vi "PushClosedSet.vi"(9 "Novo nó":dbl[](array[numeric]), 10 "ClosedSet":dbl[][](array[numeric])) -> (2 "NewClosedSet":dbl[][](array[numeric]))   [LabVIEW 2016]
panel:
  # "x"
  # "id"
  # "y"
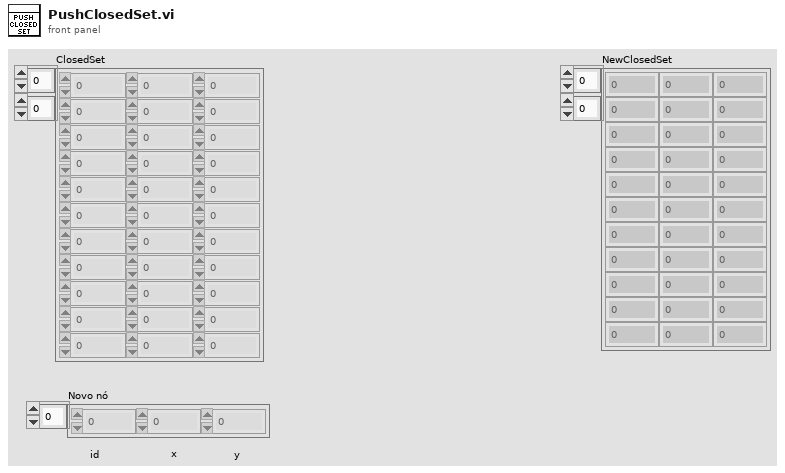
[diagram p1: front panel]
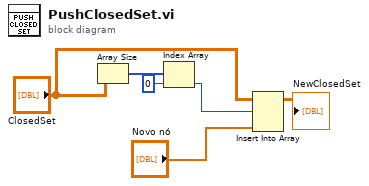
[diagram p0: block diagram]
diagram:
  n1 = Array Size(array="ClosedSet") -> (size(s)=w6:i32[])
  n2 = Index Array(array=w6, index=0) -> (element=w4:i32)
  n3 = Insert Into Array(array="ClosedSet", index (row)=w4, new element="Novo nó") -> (→"NewClosedSet":dbl[][])  [unwired: 1 in]
